vi "RingFinger.vi"(1 "Limit Switch Pressed":bool, 2 "FPGA Time":dbl, 3 "Release":bool, 4 "Intent":bool) -> ()   [LabVIEW 2013]
uses:
  <vilib>/Rock Robotics/WPI/Solenoid/WPI_SolenoidValue.ctl
  <vilib>/Rock Robotics/WPI/Solenoid/WPI_SolenoidSetEnum.vi
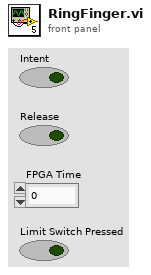
[diagram p1: front panel]
types:
  T1 = typedef "WPI_SolenoidValue.ctl" = enum16{"Off", "On", "Forward", "Reverse"}
  T2 = typedef "WPI_SolenoidDevRef.ctl" = cluster{"DevStatus":errorcluster, "Solenoid Module":T3, "Forward Solenoid Channel":T4, "Reverse Solenoid Channel":T4}
  T3 = typedef "FPGA_TypedefSolenoidModule.ctl" = enum16{"Solenoid Module 1", "Solenoid Module 2"}
  T4 = typedef "WPI_SolenoidChannel.ctl" = enum8{"Solenoid 1", "Solenoid 2", "Solenoid 3", "Solenoid 4", "Solenoid 5", "Solenoid 6", "Solenoid 7", "Solenoid 8", "Invalid"}
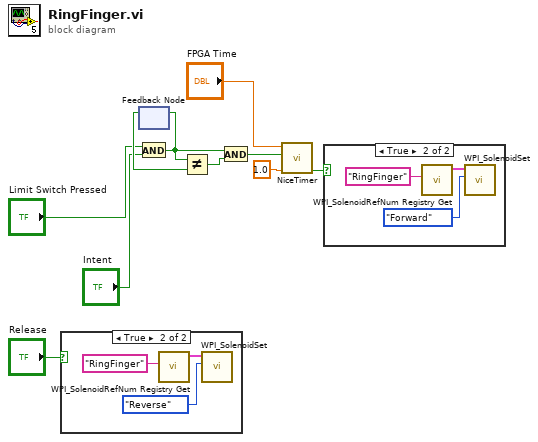
[diagram p0: block diagram]
diagram:
  n1 = case shown="True" "Release" {
    frame False {
    }
    frame True {
      n2 = call <vilib>:"WPI_SolenoidRefNum Registry Get.vi"("refnum name"="RingFinger") -> ("SolenoidDevRef"=w12:T2)  [unwired: 9 in, 1 out]
      n3 = call-poly <vilib>:"WPI_SolenoidSet.vi"("Value"=WPI_SolenoidValue."Reverse" ("t"), "SolenoidDevRef"=w12) -> ()  [unwired: 8 in, 2 out]
    }
  }
  n4 = feedback #1() -> (w5:bool)  [unwired: 1 in]
  n5 = And(x="Limit Switch Pressed", y="Intent") -> (x .and. y?=w6:bool)
  n6 = feedback-in #1(w6) -> ()
  n7 = Not Equal?(x=w6, y=w5) -> (x != y?=w4:bool)
  n8 = And(x=w6, y=w4) -> (x .and. y?=w7:bool)
  n9 = call "NiceTimer.vi"("Wait Duration"=1.0, "Reset Timer"=w7, "Current time"="FPGA Time") -> ("Single Event True"=w9:bool)  [unwired: 7 in, 1 out]
  n10 = case shown="True" w9 {
    frame False {
    }
    frame True {
      n11 = call <vilib>:"WPI_SolenoidRefNum Registry Get.vi"("refnum name"="RingFinger") -> ("SolenoidDevRef"=w15:T2)  [unwired: 9 in, 1 out]
      n12 = call-poly <vilib>:"WPI_SolenoidSet.vi"("Value"=WPI_SolenoidValue."Forward" ("t"), "SolenoidDevRef"=w15) -> ()  [unwired: 8 in, 2 out]
    }
  }
